vi "LowPressureWaxTest.vi"(0 "VI Reference In":refnum<vi>, 2 "Label":string, 11 "error in":errorcluster) -> (4 "VI Reference Out":refnum<vi>, 15 "error out":errorcluster)   [LabVIEW 2016]
uses:
  main/apis/Stimulus/ValueSignalByPathString.vi
  main/apis/Assert/AssertControlValueCompare/AssertControlValueEqual.vi
  main/apis/Assert/AssertControlValueCompare/AssertControlValueAlmostEqual.vi
  <vilib>/addons/_JKI Toolkits/Caraya/classes/Test/Test.lvclass
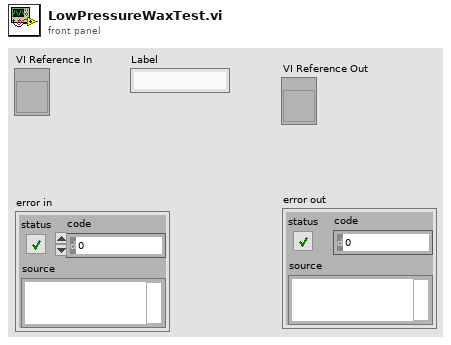
[diagram p1: front panel]
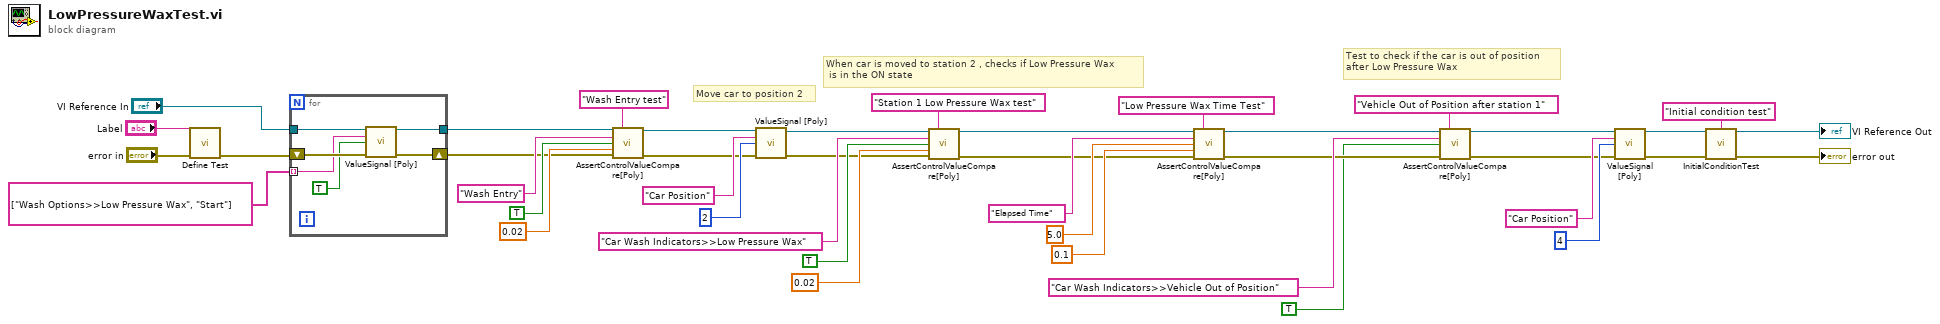
[diagram p0: block diagram]
diagram:
  # "Test to check if the car is out of position \nafter Low Pressure Wax"
  # "When car is moved to station 2 , checks if Low Pressure Wax\n is in the ON state"
  # "Move car to position 2"
  n1 = call <vilib>:"Define Test.vi"("error in (no error)"="error in", "Label (VI Title)"="Label") -> ("error out"=w38:errorcluster)  [unwired: 9 in]
  n2 = for {
    tunnel: "VI Reference In" -> [w46]
    tunnel: string[] ["Wash Options>>Low Pressure Wax", "Start"] -> [w45] mode=indexing
    shift-right: [w43] -> w31
    shift-left: w38 -> [w47]
    tunnel: [w42] -> w32
    n3 = call-poly "ValueSignal [Poly].vi"("VI Reference In"=w46, "Control Name"=w45, "Value (Signaling)"=TRUE, "error in"=w47) -> ("VI Reference Out"=w42:refnum<vi>, "error out"=w43:errorcluster)  [unwired: 10 in]
  }
  n4 = call-poly "AssertControlValueCompare[Poly].vi"("VI Reference In"=w32, "Label"="Wash Entry test", "Control Name"="Wash Entry", "Control Value"=TRUE, "Timeout(5 sec)"=0.02, "error out"=w31) -> ("VI Reference Out"=w27:refnum<vi>, "error out"=w28:errorcluster)  [unwired: 8 in]
  n5 = call-poly "ValueSignal [Poly].vi"("VI Reference In"=w27, "Control Name"="Car Position", "Value (Signaling)"=u8 2, "error in"=w28) -> ("VI Reference Out"=w11:refnum<vi>, "error out"=w12:errorcluster)  [unwired: 10 in]
  n6 = call-poly "AssertControlValueCompare[Poly].vi"("VI Reference In"=w11, "Label"="Station 1 Low Pressure Wax test", "Control Name"="Car Wash Indicators>>Low Pressure Wax", "Control Value"=TRUE, "Timeout(5 sec)"=0.02, "error out"=w12) -> ("VI Reference Out"=w18:refnum<vi>, "error out"=w19:errorcluster)  [unwired: 8 in]
  n7 = call-poly "AssertControlValueCompare[Poly].vi"("VI Reference In"=w18, "Label"="Low Pressure Wax Time Test", "Control Name"="Elapsed Time", "Control Value"=5.0, "Tolerance"=0.1, "error out"=w19) -> ("VI Reference Out"=w13:refnum<vi>, "error out"=w14:errorcluster)  [unwired: 8 in]
  n8 = call-poly "AssertControlValueCompare[Poly].vi"("VI Reference In"=w13, "Label"="Vehicle Out of Position after station 1", "Control Name"="Car Wash Indicators>>Vehicle Out of Position" ("Label"), "Control Value"=TRUE, "error out"=w14) -> ("VI Reference Out"=w5:refnum<vi>, "error out"=w4:errorcluster)  [unwired: 9 in]
  n9 = call-poly "ValueSignal [Poly].vi"("VI Reference In"=w5, "Control Name"="Car Position", "Value (Signaling)"=u8 4, "error in"=w4) -> ("VI Reference Out"=w2:refnum<vi>, "error out"=w3:errorcluster)  [unwired: 10 in]
  n10 = call "InitialConditionTest.vi"("VI Reference In"=w2, "Label"="Initial condition test", "error out"=w3) -> ("VI Reference Out"=→"VI Reference Out":refnum<vi>, "error out"=→"error out":errorcluster)  [unwired: 11 in]
